vi "PROJECT_SplashScreen_Template.vi"(11 "Allow user to close":bool) -> ()   [LabVIEW 2014, in "hse-ui.lvlib"]
uses:
  hse-ui.lvlib
  Screen_Event.ctl
  hse-application/hse-application.lvclass/hse-application.ctl
  hse-application/hse-application__GetSingleton.vi
  <vilib>/Utility/cursorutil.llb/Set Cursor (Icon Pict).vi
  <vilib>/Platform/browser.llb/Open URL in Default Browser (string).vi
  hse-application/hse-application.lvclass
panel:
  in  "Btn_Website":bool
  in  "Btn_Close":bool
  in  "Btn_Website 4":bool
  in  "Btn_Website 3":bool
  out "HSE-Lib Version:":string
  out "DQMH Version:":string
  out "Application Version:":string
  out "Application Name:":string
  out "String":string
  out "Slide":u8(slide) scale=0.0..100.0
  in  "Splash VI Event":refnum<user-event>
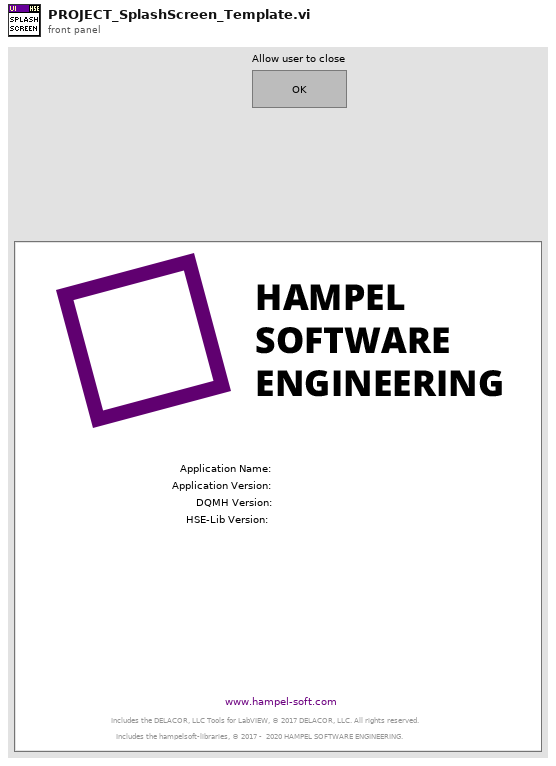
[diagram p1: front panel]
types:
  T1 = enum32{"Invalid", "Standard", "Closed", "Hidden", "Minimized", "Maximized"}
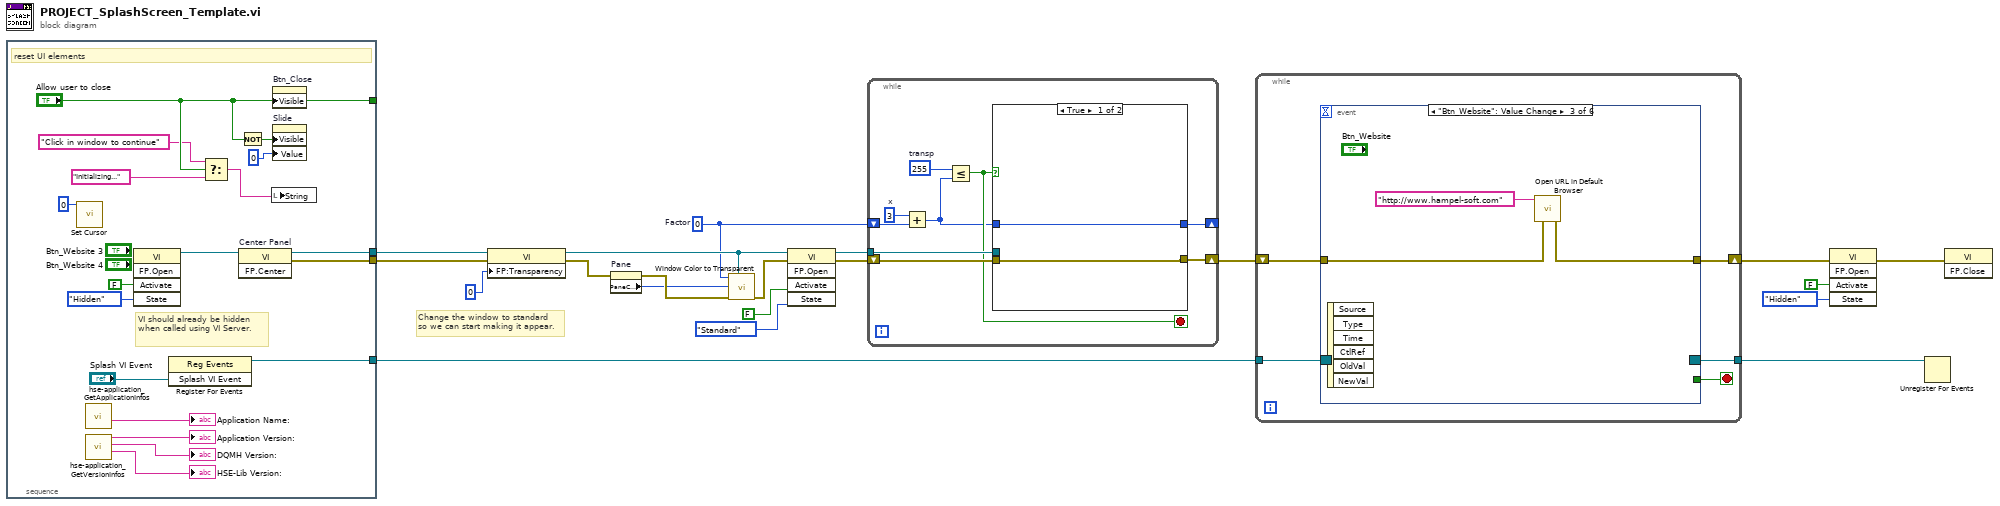
[diagram p0: block diagram]
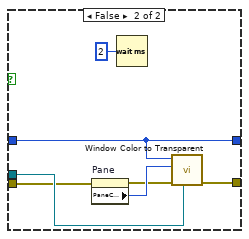
[diagram p2: hidden frame]
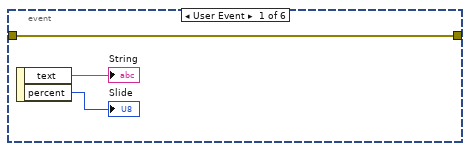
[diagram p3: hidden frame]
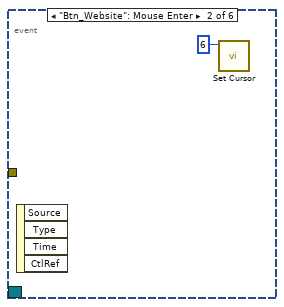
[diagram p4: hidden frame]
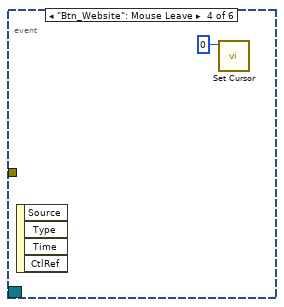
[diagram p5: hidden frame]
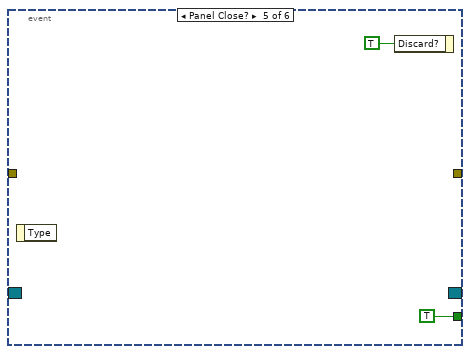
[diagram p6: hidden frame]
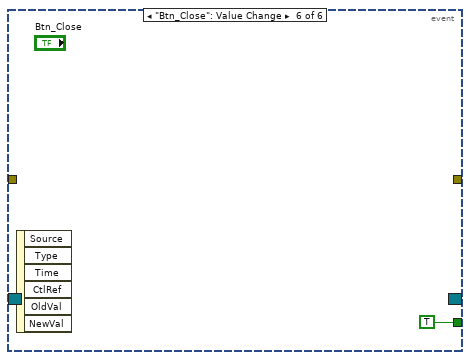
[diagram p7: hidden frame]
diagram:
  w5 = u8 0  # Factor
  # "Change the window to standard\nso we can start making it appear."
  n1 = stacked-sequence {
    tunnel: [w33] -> w17
    tunnel: [w32] -> w16
    tunnel: [w35] -> w18
    tunnel: ["Allow user to close"] -> _
    frame #0 {
      # "VI should already be hidden when called using VI Server."
      # "reset UI elements"
      n2 = call-poly <vilib>:"Set Cursor.vi"("icon"=u16 0) -> ()  [unwired: 9 in, 2 out]
      n3 = call "hse-application_GetApplicationInfos.vi"() -> ("Application Name"=→"Application Name:":string)  [unwired: 8 in, 3 out]
      n4 = call "hse-application_GetVersionInfos.vi"() -> ("HSE-LIB Version"=→"HSE-Lib Version:":string, "Framework Version"=→"DQMH Version:":string, "Application Version"=→"Application Version:":string)  [unwired: 6 in, 3 out]
      n5 = invoke class="VI" method="FP.Open"("Activate"=FALSE ("Activate?"), "State"=T1."Hidden") -> (reference out=w34:refnum<vi>)  [unwired: 3 in, 4 out]
      n6 = register-events("Splash VI Event") -> (reference out=w35:refnum<event-registration>)  [unwired: 2 in, 1 out]
      n7 = Select(t="Click in window to continue", s="Allow user to close", f="Initializing...") -> (s? t:f=w26:string)
      n8 = invoke on="Center Panel" class="VI" method="FP.Center"(reference=w34) -> (reference out=w33:refnum<vi>, error out=w32:errorcluster)  [unwired: 2 in, 1 out]
      n9 = Not(x="Allow user to close") -> (.not. x?=w31:bool)
      n10 = local write "String"(w26) -> ()
      n11 = property on="Btn_Close" class="Bool"("Visible"="Allow user to close") -> ()  [unwired: 2 in, 2 out]
      n12 = property on="Slide" class="Slide (strict)"("Visible"=w31, "Value"=u8 0 ("Slide")) -> ()  [unwired: 2 in, 2 out]
    }
  }
  n13 = property class="VI"(reference=w17, error in=w16, "FP:Transparency"=u8 0 ("t")) -> (reference out=w7:refnum<vi>, error out=w9:errorcluster)
  n14 = property on="Pane" class="Pane"(error in=w9) -> (error out=w13:errorcluster, "PaneColor"=w12:u32)  [unwired: 1 in, 1 out]
  n15 = call "Window Color to Transparent.vi"("Calling VI's reference"=w7, "error in (no error)"=w13, "Color to Replace"=w12, "Factor"=w5) -> ("error out"=w8:errorcluster)  [unwired: 7 in]
  n16 = invoke class="VI" method="FP.Open"(reference=w7, error in=w8, "Activate"=FALSE ("Activate?"), "State"=T1."Standard") -> (reference out=w11:refnum<vi>, error out=w10:errorcluster)  [unwired: 1 in, 3 out]
  n17 = while {
    shift-right: [w45] -> _
    shift-left: w5 -> [w41]
    shift-right: [w44] -> w19
    shift-left: w10 -> [w43]
    tunnel: w11 -> [w46]
    stop <- w42 stop-if-true
    w39 = u8 3  # x
    w47 = u8 255  # transp
    n18 = Add(x=w39, y=w41) -> (x+y=w40:u8)
    n19 = Less Or Equal?(x=w47, y=w40) -> (x <= y?=w42:bool)
    n20 = case shown="True" w42 {
      tunnel: w40 -> [w49 w53]
      tunnel: w46 -> [_ w54]
      tunnel: [w49 w53] -> w45
      tunnel: [w48 w52] -> w44
      tunnel: w43 -> [w48 w51]
      frame True {
      }
      frame False {
        n21 = property on="Pane" class="Pane"(error in=w51) -> (error out=w55:errorcluster, "PaneColor"=w56:u32)  [unwired: 1 in, 1 out]
        n22 = Wait (ms)(milliseconds to wait=u32 2) -> ()  [unwired: 1 out]
        n23 = call "Window Color to Transparent.vi"("Calling VI's reference"=w54, "error in (no error)"=w55, "Color to Replace"=w56, "Factor"=w53) -> ("error out"=w52:errorcluster)  [unwired: 7 in]
      }
    }
  }
  n24 = while {
    shift-right: [w61] -> w2
    shift-left: w19 -> [w59]
    tunnel: [w58] -> w20
    tunnel: w18 -> [w57]
    stop <- w60 stop-if-true
    n25 = event shown="[2] \"Btn_Website\": Value Change" {
      selector: w57 -> [_ _ _ _ _ _]
      dyn-events: [_ _ _ _ _ _] -> w58
      timeout: _ -> [_ _ _ _ _ _]
      tunnel: w59 -> [w64 _ w66 _ _ _]
      tunnel: [w64 _ w67 _ _ _] -> w61
      tunnel: [_ _ _ _ TRUE ("Close") TRUE ("Close")] -> w60
      event User Event {
        n26 = event-data() -> ("text"=→"String":string, "percent"=→"Slide":i32)  [unwired: 1 in]
      }
      event "Btn_Website": Mouse Enter {
        n27 = event-data() -> ()  [unwired: 1 in, 4 out]
        n28 = call-poly <vilib>:"Set Cursor.vi"("icon"=u16 6) -> ()  [unwired: 9 in, 2 out]
      }
      event "Btn_Website": Value Change {
        n29 = event-data() -> ()  [unwired: 1 in, 6 out]
        n30 = call-poly <vilib>:"Open URL in Default Browser.vi"("error in (no error)"=w66, "URL"="http://www.hampel-soft.com" ("Link")) -> ("error out"=w67:errorcluster)  [unwired: 4 in, 1 out]
      }
      event "Btn_Website": Mouse Leave {
        n31 = event-data() -> ()  [unwired: 1 in, 4 out]
        n32 = call-poly <vilib>:"Set Cursor.vi"("icon"=u16 0) -> ()  [unwired: 9 in, 2 out]
      }
      event Panel Close? {
        n33 = event-data() -> ()  [unwired: 1 in, 1 out]
        n34 = event-data("Discard?"=TRUE) -> ()  [unwired: 1 in, 1 out]
      }
      event "Btn_Close": Value Change {
        n35 = event-data() -> ()  [unwired: 1 in, 6 out]
      }
    }
  }
  n36 = invoke class="VI" method="FP.Open"(error in=w2, "Activate"=FALSE ("Activate?"), "State"=T1."Hidden") -> (error out=w1:errorcluster)  [unwired: 2 in, 4 out]
  n37 = Unregister For Events(event registration refnum=w20) -> ()  [unwired: 1 in, 1 out]
  n38 = invoke class="VI" method="FP.Close"(error in=w1) -> ()  [unwired: 2 in, 3 out]
